vi "00_CreateLOGfile.vi"(11 "LOG file":path) -> (3 "refnum out":refnum<file>)   [LabVIEW 2017]
uses:
  <vilib>/Utility/error.llb/whitespace.ctl
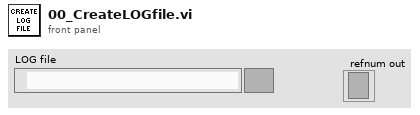
[diagram p1: front panel]
types:
  T1 = typedef "whitespace.ctl" = u16
  T2 = enum16{"open", "replace", "create", "open or create", "replace or create", "replace or create with confirmation"}
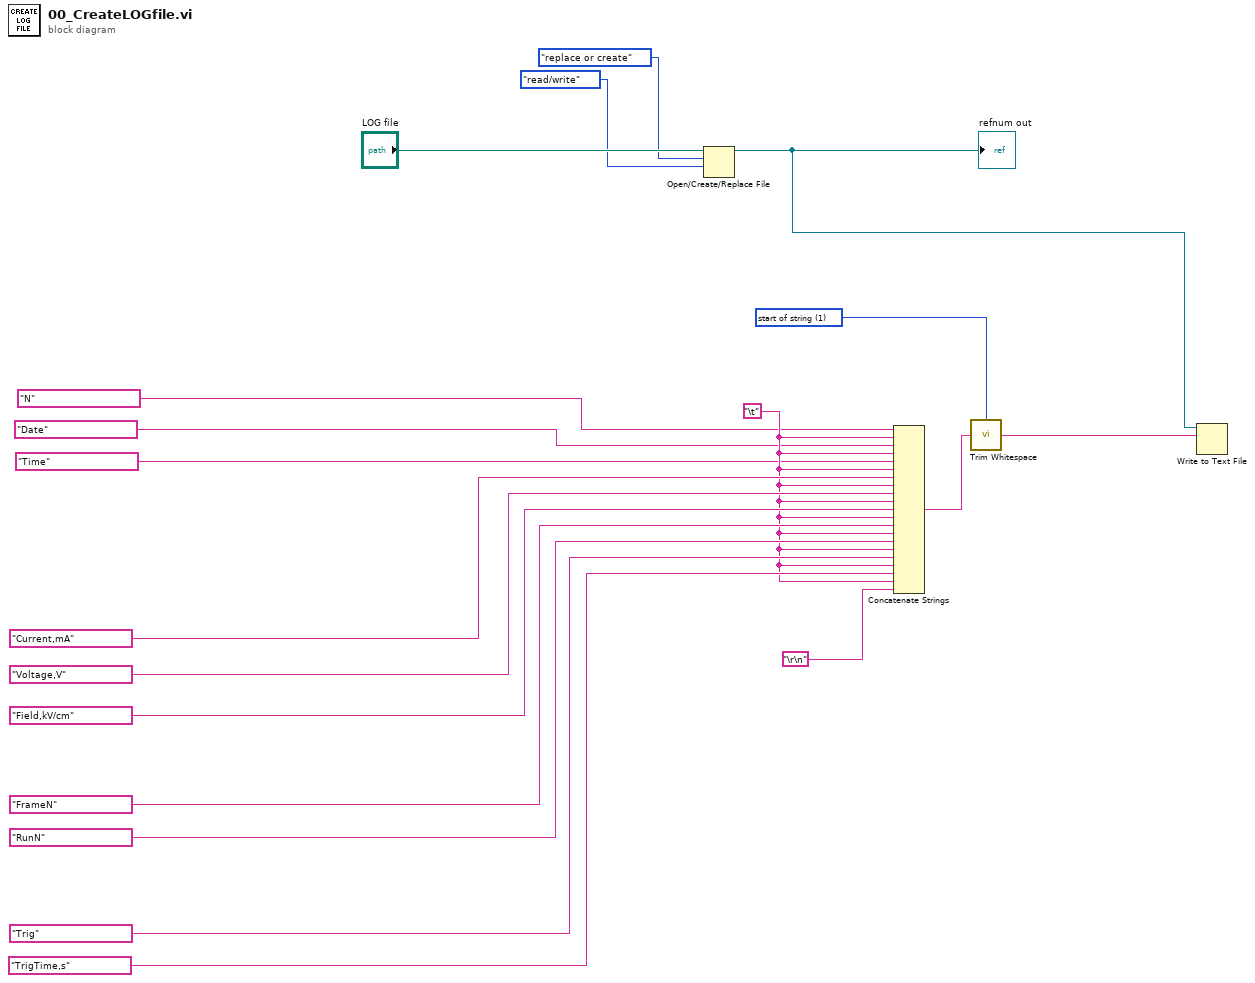
[diagram p0: block diagram]
diagram:
  w5 = "\t"
  w15 = T1 1 items=["both", "start of string", "end of string"] ("location (both)")
  n1 = Open/Create/Replace File(file path (use dialog)="LOG file", operation (0:open)=T2."replace or create", access (0:read/write)=enum16{"read/write", "read-only", "write-only"}."read/write") -> (refnum out=w8:refnum<file>)  [unwired: 3 in, 2 out]
  "refnum out" <- w8
  n2 = Concatenate Strings("N" ("string"), w5, "Date" ("string"), w5, "Time" ("string"), w5, "Current,mA" ("string"), w5, "Voltage,V" ("string"), w5, "Field,kV/cm" ("string"), w5, "FrameN" ("string"), w5, "RunN" ("string"), w5, "Trig" ("string"), w5, "TrigTime,s" ("string"), w5, "\r\n") -> (w16:string)
  n3 = call <vilib>:"Trim Whitespace.vi"("string"=w16, "location (both)"=w15) -> ("trimmed string"=w7:string)
  n4 = Write to Text File(file (use dialog)=w8, text=w7) -> ()  [unwired: 2 in, 3 out]
